vi "Timer.vi"(8 "entrée d'erreur":errorcluster caption="entrée d'erreur (pas d'erreur)", 10 "Timer (Sec)":dbl, 11 "State":T1) -> (0 "sortie d'erreur":errorcluster, 2 "Elapsed":dbl, 3 "Elapsed?":bool)   [LabVIEW 2021]
doc: "This is the Timer VI with the states:\nStart, Elapsed Time and Pause.\nDesigne Patter: FGV"
uses:
  Controls/Time.ctl
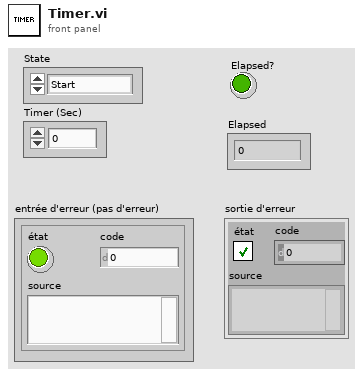
[diagram p1: front panel]
types:
  T1 = typedef "Time.ctl" = enum16{"Start", "Elapsed", "Pause", "int"}
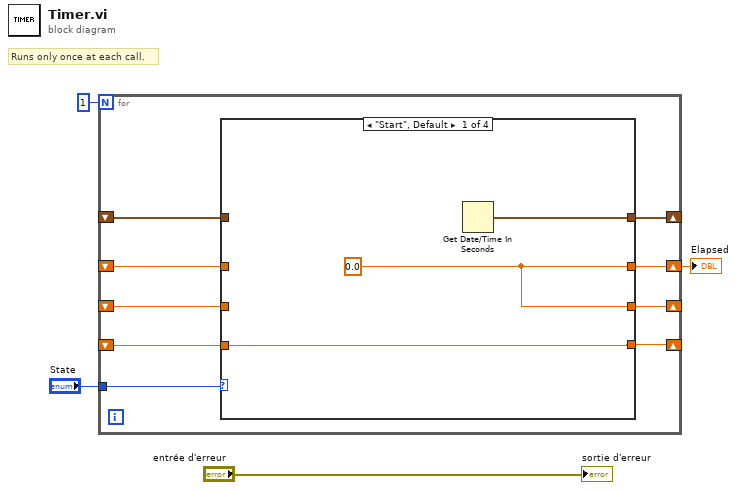
[diagram p0: block diagram]
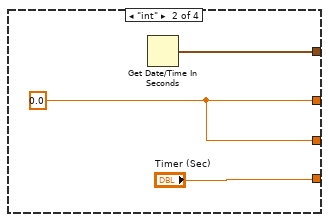
[diagram p2: hidden frame]
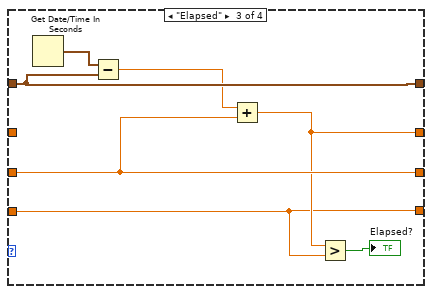
[diagram p3: hidden frame]
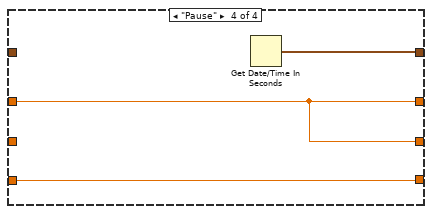
[diagram p4: hidden frame]
diagram:
  # "Runs only once at each call."
  n1 = for {
    N: 1 -> [_]
    tunnel: "State" -> [w13]
    shift-right: [w12] -> _
    shift-left: _ -> [w11]
    shift-right: [w10] -> w2
    shift-left: _ -> [w7]
    shift-right: [w9] -> _
    shift-left: _ -> [w6]
    shift-right: [w8] -> _
    shift-left: _ -> [w5]
    n2 = case shown="\"Start\", Default" w13 {
      tunnel: [w16 w19 w24 w29] -> w12
      tunnel: w11 -> [_ _ w24 _]
      tunnel: [w15 w18 w21 w28] -> w10
      tunnel: [w15 w18 w22 w28] -> w9
      tunnel: [w14 "Timer (Sec)" w20 w27] -> w8
      tunnel: w7 -> [_ _ _ w28]
      tunnel: w6 -> [_ _ w22 _]
      tunnel: w5 -> [w14 _ w20 w27]
      frame "Start", Default {
        w15 = 0.0
        n3 = Get Date/Time In Seconds() -> (seconds since 1Jan1904=w16:timestamp)
      }
      frame "int" {
        w18 = 0.0
        n4 = Get Date/Time In Seconds() -> (seconds since 1Jan1904=w19:timestamp)
      }
      frame "Elapsed" {
        n5 = Get Date/Time In Seconds() -> (seconds since 1Jan1904=w26:timestamp)
        n6 = Subtract(x=w26, y=w24) -> (x-y=w23:dbl)
        n7 = Add(x=w23, y=w22) -> (x+y=w21:dbl)
        n8 = Greater?(x=w21, y=w20) -> (0:→"Elapsed?":bool)
      }
      frame "Pause" {
        n9 = Get Date/Time In Seconds() -> (seconds since 1Jan1904=w29:timestamp)
      }
    }
  }
  "Elapsed" <- w2
  "sortie d'erreur" <- "entrée d'erreur"
